vi "sample changer vars.vi"() -> ()   [LabVIEW 2016]
panel:
  in  "stop":bool
  in  "wheel readback":dbl
  in  "use1":string[](array[string])
  in  "stop random sample change":bool
  in  "start random sample change":bool
  in  "set vent system":bool
  in  "set sc open":bool
  in  "set sc close":bool
  in  "set rod up1":bool
  in  "set rod down":bool
  in  "set retract out":bool
  in  "set retract in":bool
  in  "set pump out system":bool
  in  "set insert out":bool
  in  "set insert in":bool
  in  "set cold cathode on":bool
  in  "set cold cathode off":bool
  in  "sc control":string
  in  "sample number":i16
  in  "rotate wheel":bool
  in  "rod up shared":bool
  in  "read sc gv open":bool
  in  "read sc gv closed":bool
  in  "read rod up":bool
  in  "read rod  down":bool
  in  "read retract out":bool
  in  "read retract in":bool
  in  "read insert out":bool
  in  "read insert in":bool
  in  "position":dbl
  in  "listofstuff":string[](array[string])
  in  "indextest":i16
  in  "index2":string
  in  "ig2":string
  in  "ig1":string
  in  "feedback":string
  in  "end test":bool
  in  "count":dbl
  in  "convectron":string
  in  "cold cathode on":bool
  in  "cold cathode off":bool
  in  "cold cathode":dbl
  in  "change sample":bool
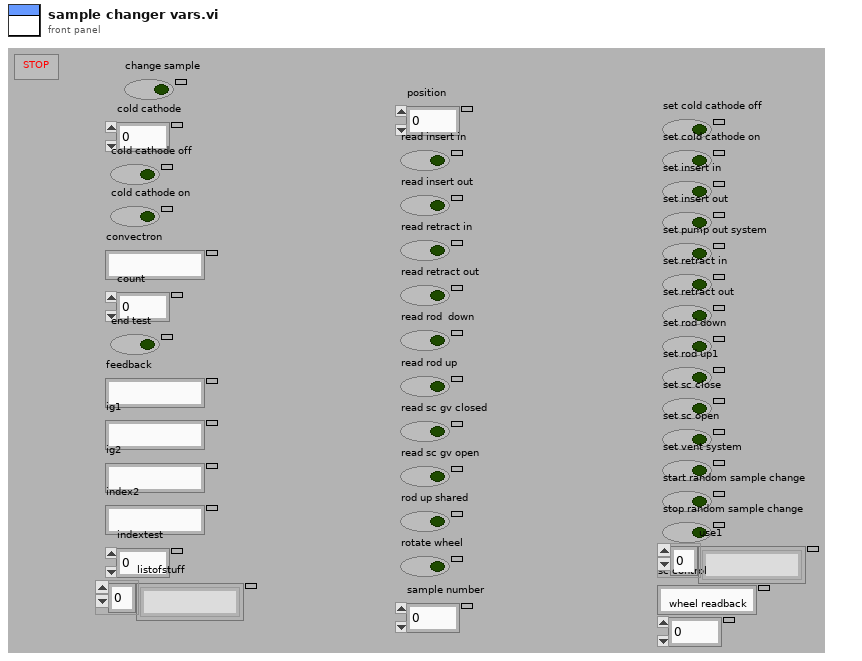
[diagram p1: front panel]
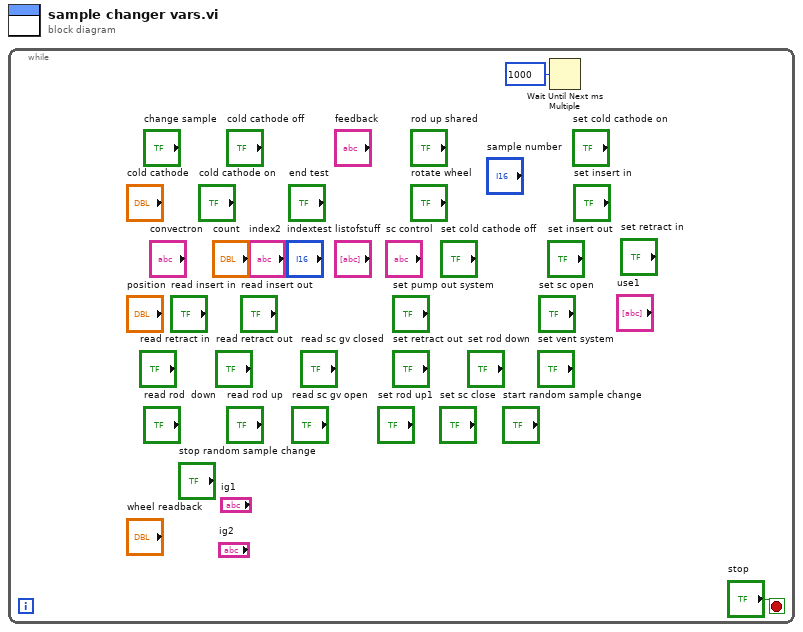
[diagram p0: block diagram]
diagram:
  n1 = while {
    stop <- "stop" stop-if-true
    n2 = Wait Until Next ms Multiple(millisecond multiple=u32 1000) -> ()  [unwired: 1 out]
  }
